vi "Swap Refs.vi"(8 "error in (no error)":errorcluster, 10 "Old Ref":refnum<class "Alicat.lvclass">, 11 "New Ref":refnum<class "Alicat.lvclass">) -> (0 "error out":errorcluster, 3 "Alicat out":refnum<class "Alicat.lvclass">)   [LabVIEW 2015, in "Alicat.lvlib" / "Alicat.lvclass"]
doc: "Swap Refs is used when recasting a device. If the user initializes some of the properties of the particular Alicat device prior to calling the recast VI, then those properties will necessarily be lost if they are not explicitly preserved. If this is called and the generic implementation is all that is available, then the device will behave as if nothing happened."
uses:
  Alicat.lvclass
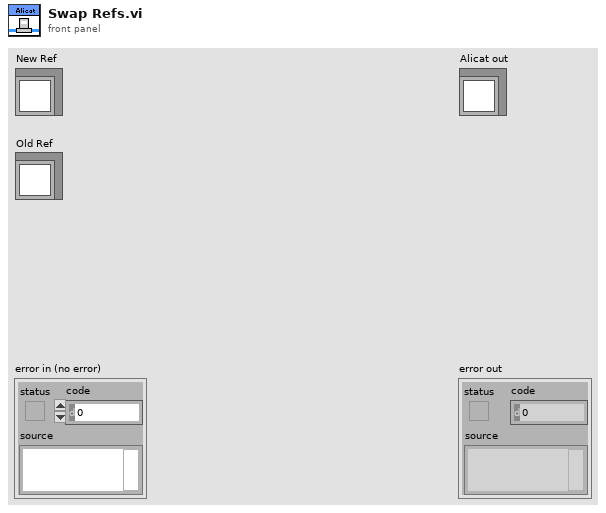
[diagram p1: front panel]
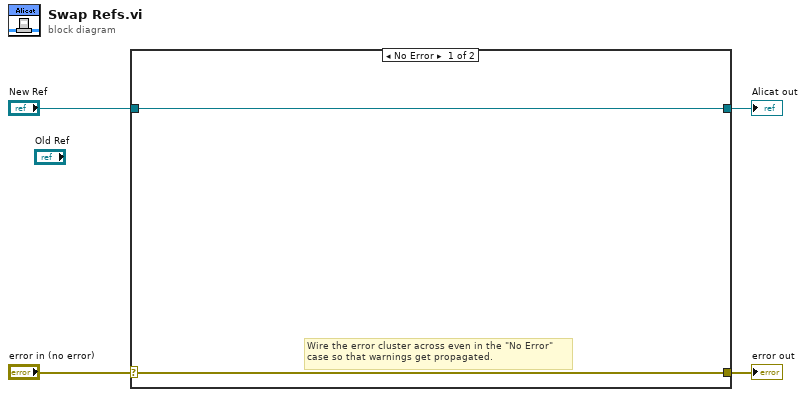
[diagram p0: block diagram]
diagram:
  n1 = case shown="No Error" "error in (no error)" {
    selector: "error in (no error)" -> [w5 w8]
    tunnel: [w5 w8] -> w3
    tunnel: [w6 w7] -> w1
    tunnel: "New Ref" -> [w6 w7]
    frame No Error {
      # "Wire the error cluster across even in the \"No Error\"\ncase so that warnings get propagated."
    }
    frame Error {
    }
  }
  "error out" <- w3
  "Alicat out" <- w1
